vi "ObtainMessageQueue.vi"(7 "max queue size (-1, unlimited)":i32, 8 "error in (no error)":errorcluster) -> (0 "error out":errorcluster, 3 "MessageQueue":refnum<queue>)   [LabVIEW 2015]
doc: "Erstellt eine Queue mit \"MessageCluster\" als Datentyp der Queue."
uses:
  TypeDefs/MessageCluster.ctl
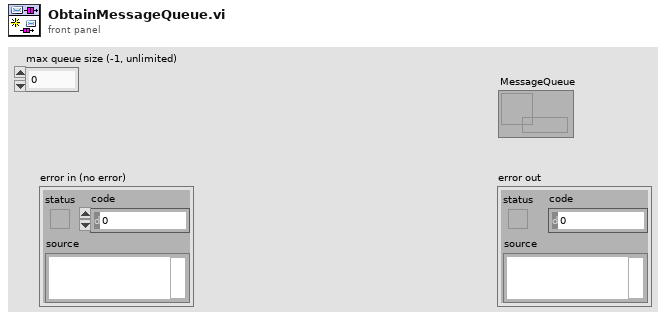
[diagram p1: front panel]
types:
  T1 = typedef "MessageCluster.ctl" = cluster{"Message":string, "MessageData":variant}
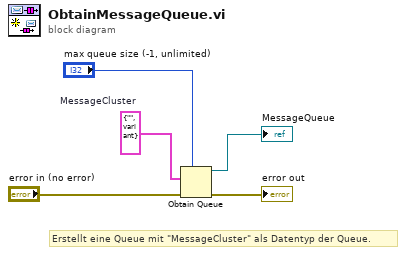
[diagram p0: block diagram]
diagram:
  w5 = T1 {"Message"="", "MessageData"=variant}  # MessageCluster
  # "Erstellt eine Queue mit \"MessageCluster\" als Datentyp der Queue."
  n1 = Obtain Queue(max queue size (-1, unlimited)="max queue size (-1, unlimited)", element data type=w5, error in (no error)="error in (no error)") -> (queue out=→"MessageQueue":refnum<queue>, error out=→"error out":errorcluster)  [unwired: 2 in, 1 out]
